vi "Flatten.vi"(8 "error in (no error)":errorcluster, 10 "Pretty Print?":bool, 11 "JSON Object in":refnum<class "JSON Object.lvclass">) -> (0 "error out":errorcluster, 2 "<JSON>":string)   [LabVIEW 2020, in "Library Commun.lvlib" / "JSON Object.lvclass"]
doc: "Converts an <b>JSON Object</b> into <b>String</b>. Use <b>Pretty Print?</b> to auto-indent and distribute the string over different lines.\n\nCopyright 2012 James David Powell, Shaun Rumbell and Ton Plomp\nMore information on http://lavag.org/topic/16217-cr-json-labview"
uses:
  JSON Object.lvclass
  JSON Object.lvclass/JSON Object.ctl
  JSON Value/JSON Value.lvclass
  support/JSON support.lvlib
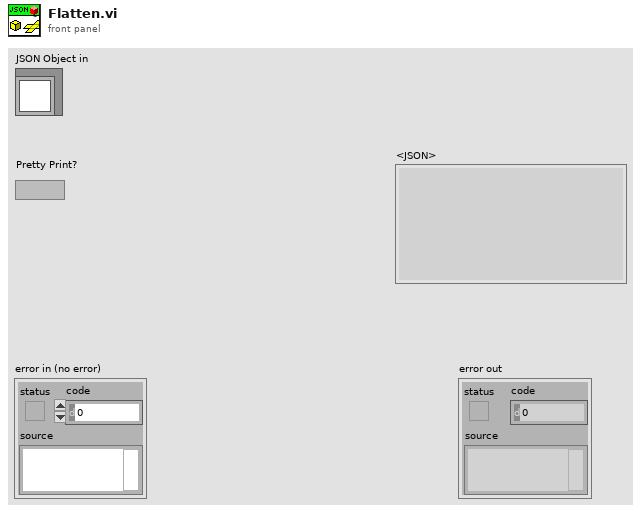
[diagram p1: front panel]
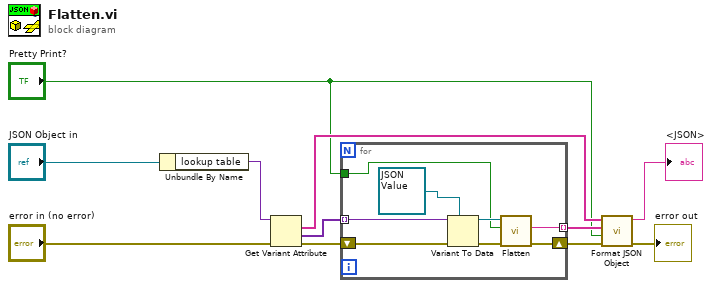
[diagram p0: block diagram]
diagram:
  n1 = Unbundle By Name("JSON Object in") -> ("lookup table"=w10:variant)
  n2 = Get Variant Attribute(Variant=w10, error in="error in (no error)") -> (names=w9:string[], values=w5:variant[], error out=w4:errorcluster)  [unwired: 2 in, 1 out]
  n3 = for {
    tunnel: w5 -> [w17] mode=indexing
    shift-right: [w14] -> w3
    shift-left: w4 -> [w16]
    tunnel: [w13] -> w2 mode=indexing
    tunnel: "Pretty Print?" -> [w12]
    n4 = Variant To Data(error in=w16, type=refnum<class "JSON Value.lvclass"> refnum ("JSON Value.lvclass"), Variant=w17) -> (data=w19:refnum<class "JSON Value.lvclass">, error out=w15:errorcluster)
    n5 = call-dynamic "Flatten.vi"("error in (no error)"=w15, "Pretty Print?"=w12, "JSON Value in"=w19) -> ("error out"=w14:errorcluster, "<JSON>"=w13:string)  [unwired: 7 in]
  }
  n6 = call "Format JSON Object.vi"("error in (no error)"=w3, "Pretty Print?"="Pretty Print?", "JSON elements"=w2, "Names"=w9) -> ("error out"=→"error out":errorcluster, "JSON Object Text out"=→"<JSON>":string)  [unwired: 6 in]
